vi "Test Alignement.vi"() -> ()   [LabVIEW 2021]
uses:
  <vilib>/Utility/miscctls.llb/LVRectTypeDef.ctl
  <vilib>/Utility/miscctls.llb/LVPositionTypeDef.ctl
panel:
  in  "Close":bool
  in  "Undock":bool
  in  "Settings":bool
  in  "Minimize":bool
  in  "Maximize 2":bool
  in  "Maximize":bool
  in  "Collapse":bool
  in  "Border":i32
  out "Content Area Rect":T1
  out "Zones Rectangles":T2(array[cluster])
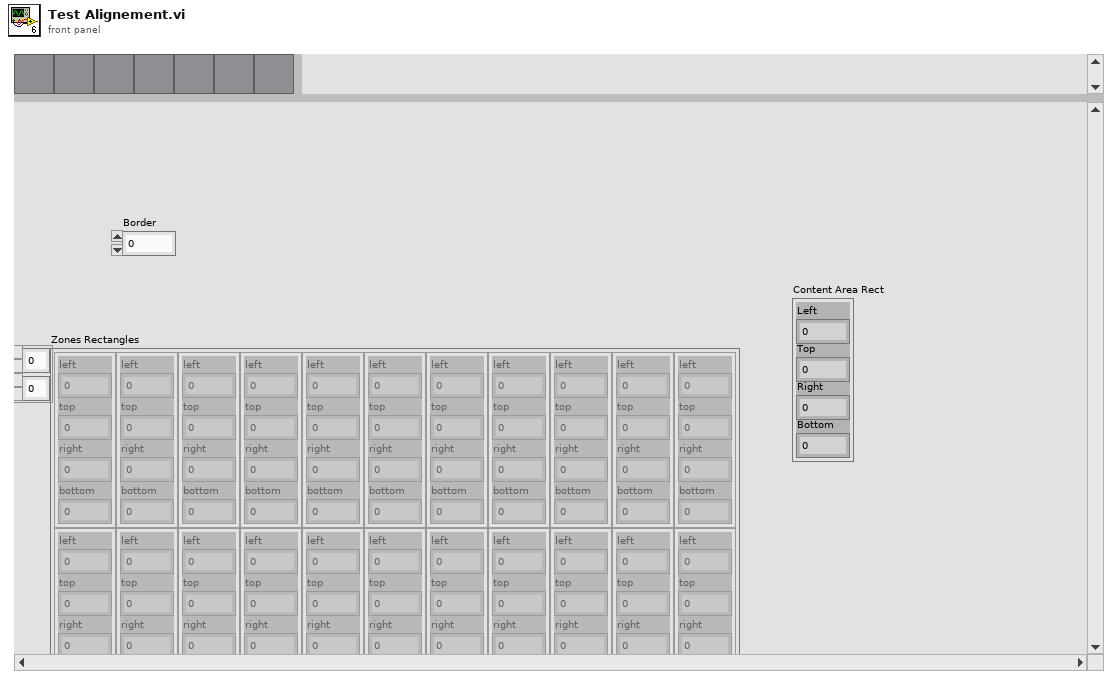
[diagram p1: front panel]
types:
  T1 = typedef "LVRectTypeDef.ctl" = cluster{"Left":i16, "Top":i16, "Right":i16, "Bottom":i16}
  T2 = cluster{"left":i16, "top":i16, "right":i16, "bottom":i16}[][]
  T3 = cluster{"left":i16, "top":i16, "right":i16, "bottom":i16}
  T4 = cluster{"left":i16, "top":i16, "right":i16, "bottom":i16}[]
  T5 = typedef "LVPositionTypeDef.ctl" = cluster{"Left":i32, "Top":i32}
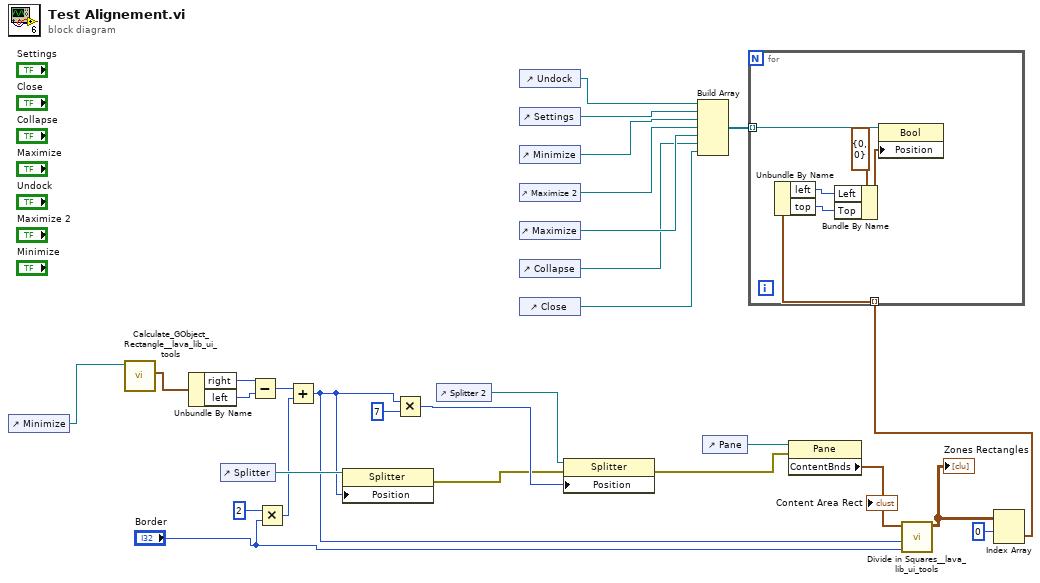
[diagram p0: block diagram]
diagram:
  n1 = control-ref of="Minimize"() -> (w25:refnum<vi>)
  n2 = call <vilib>:"Calculate_GObject_Rectangle__lava_lib_ui_tools.vi"("GObject ref"=w25) -> ("Rectangle"=w28:T3)  [unwired: 8 in, 2 out]
  n3 = Unbundle By Name(w28) -> ("right"=w27:i16, "left"=w26:i16)
  n4 = control-ref of="Splitter"() -> (w24:refnum<vi>)
  n5 = Subtract(x=w27, y=w26) -> (x-y=w22:i16)
  n6 = Multiply(x=2, y="Border") -> (x*y=w3:i32)
  n7 = Add(x=w22, y=w3) -> (x+y=w4:i32)
  n8 = property class="Splitter"(reference=w24, "Position"=w4) -> (error out=w10:errorcluster)  [unwired: 1 in, 1 out]
  n9 = Multiply(x=w4, y=i16 7) -> (x*y=w21:i32)
  n10 = control-ref of="Splitter 2"() -> (w20:refnum<vi>)
  n11 = control-ref of="Undock"() -> (w19:refnum<vi>)
  n12 = control-ref of="Settings"() -> (w18:refnum<vi>)
  n13 = control-ref of="Minimize"() -> (w17:refnum<vi>)
  n14 = control-ref of="Maximize 2"() -> (w16:refnum<vi>)
  n15 = control-ref of="Maximize"() -> (w15:refnum<vi>)
  n16 = control-ref of="Collapse"() -> (w14:refnum<vi>)
  n17 = control-ref of="Close"() -> (w13:refnum<vi>)
  n18 = property class="Splitter"(reference=w20, error in=w10, "Position"=w21) -> (error out=w8:errorcluster)  [unwired: 1 out]
  n19 = Build Array(w19, w18, w17, w16, w15, w14, w13) -> (w12:refnum<vi>[])
  n20 = control-ref of="Pane"() -> (w9:refnum<vi>)
  n21 = property class="Pane"(reference=w9, error in=w8) -> ("ContentBnds"=w7:T1)  [unwired: 2 out]
  "Content Area Rect" <- w7
  n22 = call <vilib>:"Divide in Squares__lava_lib_ui_tools.vi"("Border (2)"="Border", "Width (48)"=w4, "Rectangle"=w7) -> ("Zones Rectangles"=w11:T2)  [unwired: 5 in, 3 out]
  "Zones Rectangles" <- w11
  n23 = Index Array(array=w11, index (row)=0) -> (element=w5:T4)  [unwired: 1 in]
  n24 = for {
    tunnel: w12 -> [w34] mode=indexing
    tunnel: w5 -> [w33] mode=indexing
    n25 = Unbundle By Name(w33) -> ("left"=w30:i16, "top"=w29:i16)
    n26 = Bundle By Name(cluster=T5 {"Left"=0, "Top"=0} ("Position"), "Left"=w30, "Top"=w29) -> (w31:T5)
    n27 = property class="Bool"(reference=w34, "Position"=w31) -> ()  [unwired: 1 in, 2 out]
  }
